vi "Move Marker.vi"(0 "VISA resource name":refnum<visa-resource-name>, 5 "Marker (0:Marker to Center)":i32(ring) items=["Marker to Center", "Marker to Reference", "Peak to Center", "Peak to Reference", "All OFF"], 11 "error in (no error)":errorcluster) -> (4 "VISA resource name out":refnum<visa-resource-name>, 15 "error out":errorcluster)   [LabVIEW 2020, in "Anritsu Signal Analyzer Series.lvlib"]
doc: "Sets the marker frequency to the center frequency.\nSets the marker level to the reference level.\nSets the maximum peak point to the center frequency.\nSets the maximum peak point to the reference level."
uses:
  Anritsu Signal Analyzer Series.lvlib
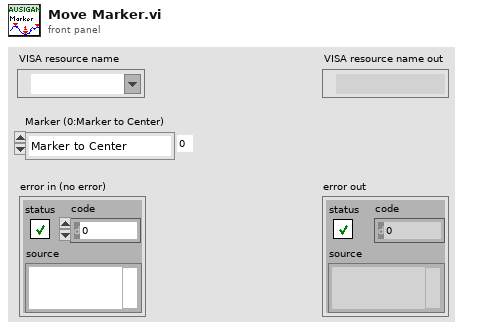
[diagram p1: front panel]
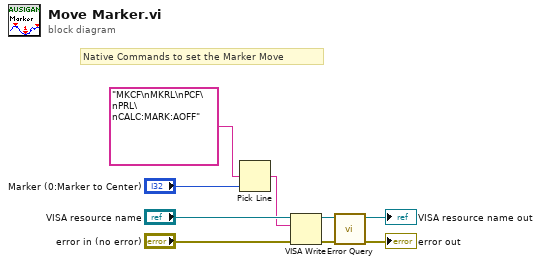
[diagram p0: block diagram]
diagram:
  # "Native Commands to set the Marker Move"
  n1 = Pick Line(multi-line string="MKCF\nMKRL\nPCF\nPRL\nCALC:MARK:AOFF" ("_Command"), line index="Marker (0:Marker to Center)") -> (output string=w2:string)  [unwired: 1 in]
  n2 = VISA Write(VISA resource name="VISA resource name", write buffer=w2, error in (no error)="error in (no error)") -> (VISA resource name out=w4:refnum<visa-resource-name>, error out=w5:errorcluster)  [unwired: 1 out]
  n3 = call "Error Query.vi"("error in (no error)"=w5, "VISA resource name"=w4) -> ("error out"=→"error out":errorcluster, "VISA resource name out"=→"VISA resource name out":refnum<visa-resource-name>)  [unwired: 6 in, 2 out]
